vi "HAL camera stop.vi"   [LabVIEW 2011]
uses:
  Cascade-specific globals.vi
  Camera/camera globals.vi
types:
  T1 = cluster{"Camera Handle":u32, "Pulser Handle":u32, "File Handle":u32, "Display Handle":u32, "Image Handle":u32}
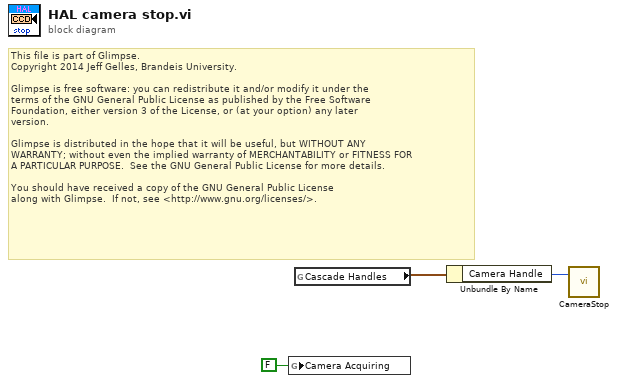
[diagram p0: block diagram]
diagram:
  # "This file is part of Glimpse. \nCopyright 2014 Jeff Gelles, Brandeis University.    \n\nGlimpse is free software: you can redistribute it and/or modify it under the \nterms of the GNU General Public License as published by the Free Software \nFoundation, either version 3 of the License, or (at your option) any later \nversion.\n\nGlimpse is distributed in the hope that it will be useful, but WITHOUT ANY \nWARRANTY; without even the implied warranty of MERCHANTABILITY or FITNESS FOR \nA PARTICULAR PURPOSE.  See the GNU General Public License for more details.\n\nYou should have received a copy of the GNU General Public License\nalong with Glimpse.  If not, see <http://www.gnu.org/licenses/>."
  n1 = global write "camera globals.vi" "Camera Acquiring"(FALSE ("Camera Acquiring")) -> ()
  n2 = global read "Cascade-specific globals.vi" "Cascade Handles"() -> (w3:T1)
  n3 = Unbundle By Name(w3) -> ("Camera Handle"=w2:u32)
  n4 = call <userlib>:"CameraStop.vi"("Camera Handle"=w2) -> ()  [unwired: 1 in, 2 out]
